vi "LinTabelle zusammenbauen.vi"(8 "error in (no error)":errorcluster caption="Fehler (Eingang, kein Fehler)", 11 "Eingabetabelle":T1) -> (0 "error out":errorcluster caption="Fehler (Ausgang)", 1 "XY-Graph":cluster{dbl[], dbl[]}[](array[cluster]), 2 "Eingabetabelle behandelt":string[][](array[string]), 3 "LIN Ausgabetabelle":string[][](table))   [LabVIEW 2020, in "Linearisierung v2.lvlib"]
uses:
  Linearisierung v2.lvlib
  Eingabetabelle.ctl
panel:
  # "Tabelle:\n0.....Sollwert\n1.....Istwert\n2.....Rohwert\n3.....linearisiert\n4.....abs.Fehler ppm\n5.....Fehler in %\n6.....Deviation\n7.....Temp.Messzelle\n8.....Druck Messzelle\n9.....abs.Fehler ppm linearisiert\n10....Fehler in % linearisiert\n11....abs.Fehler ppm EPA\n12....Fehler in % EPA\n13....abs.Fehler ppm Rohwert\n14....Fehler in % Rohwert"
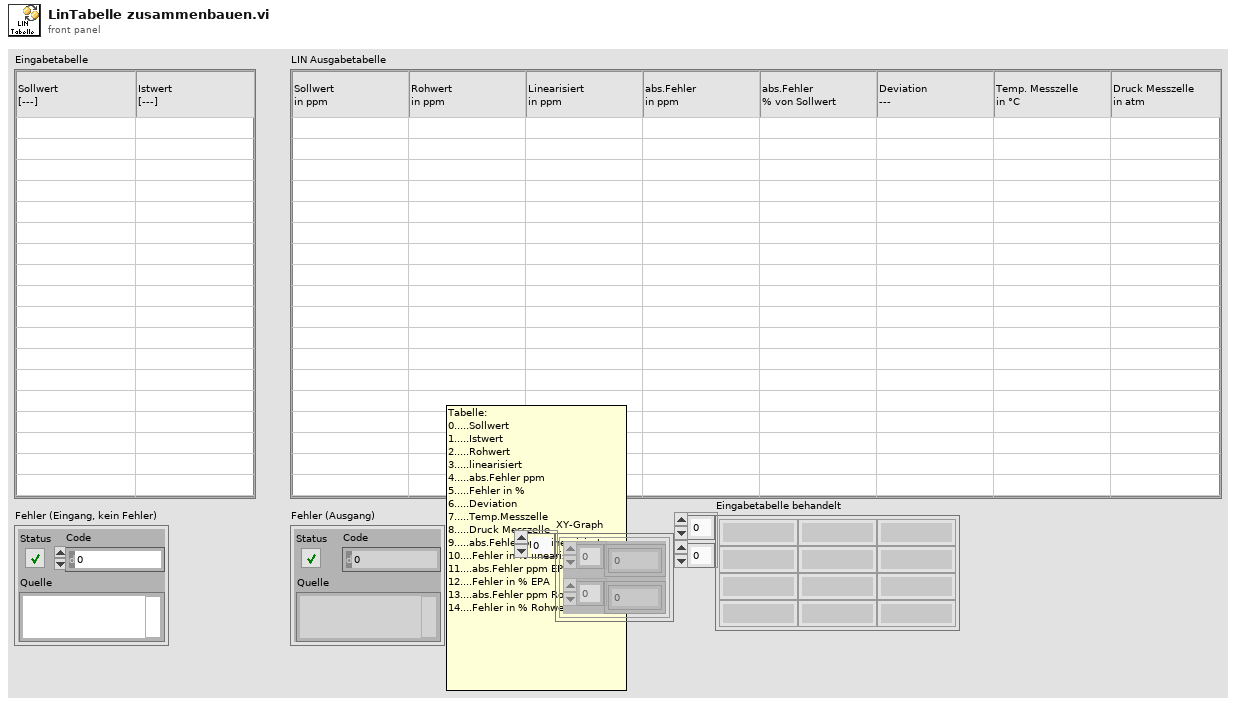
[diagram p1: front panel]
types:
  T1 = typedef "Linearisierung v2.lvlib/Eingabetabelle.ctl" = string[][]
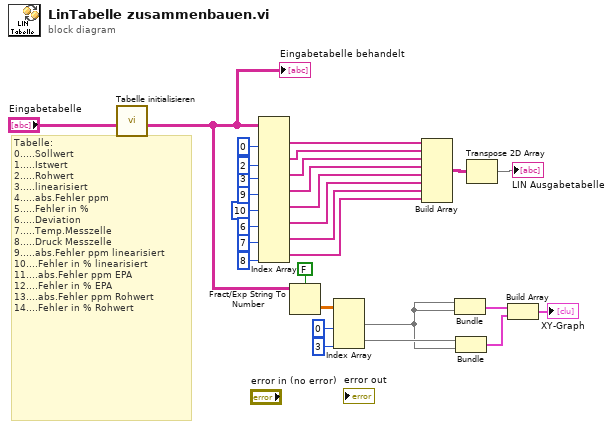
[diagram p0: block diagram]
diagram:
  # "Tabelle:\n0.....Sollwert\n1.....Istwert\n2.....Rohwert\n3.....linearisiert\n4.....abs.Fehler ppm\n5.....Fehler in %\n6.....Deviation\n7.....Temp.Messzelle\n8.....Druck Messzelle\n9.....abs.Fehler ppm linearisiert\n10....Fehler in % linearisiert\n11....abs.Fehler ppm EPA\n12....Fehler in % EPA\n13....abs.Fehler ppm Rohwert\n14....Fehler in % Rohwert"
  n1 = call "Tabelle initialisieren.vi"("Neue Tabelle"="Eingabetabelle") -> ("Tabelle"=w2:string[][])  [unwired: 10 in]
  "Eingabetabelle behandelt" <- w2
  n2 = Index Array(array=w2, index (col) #1=0 ("Deaktivierter Index (Spalte)"), index (col) #2=2 ("Index (Spalte)"), index (col) #3=3 ("Index (Spalte)"), index (col) #4=9 ("Index (Spalte)"), index (col) #5=10 ("Index (Spalte)"), index (col) #6=6 ("Index (Spalte)"), index (col) #7=7 ("Index (Spalte)"), index (col) #8=8 ("Index (Spalte)")) -> (element #1=w29:string[], element #2=w28:string[], element #3=w24:string[], element #4=w21:string[], element #5=w20:string[], element #6=w16:string[], element #7=w15:string[], element #8=w14:string[])  [unwired: 8 in]
  n3 = Fract/Exp String To Number(use system decimal point (T)=FALSE ("Systemdezimalzeichen verwenden (T)"), string=w2) -> (number=w6:dbl[][])  [unwired: 2 in, 1 out]
  n4 = Index Array(array=w6, index (col) #1=0 ("Deaktivierter Index (Spalte)"), index (col) #2=3 ("Index (Spalte)")) -> (element #1=w9:dbl[], element #2=w10:dbl[])  [unwired: 2 in]
  n5 = Build Array(w29, w28, w24, w21, w20, w16, w15, w14) -> (w13:string[][])
  n6 = Bundle(w9, w9) -> (w4:cluster{dbl[], dbl[]})  [unwired: 1 in]
  n7 = Bundle(w10, w9) -> (w5:cluster{dbl[], dbl[]})  [unwired: 1 in]
  n8 = Transpose 2D Array(2D array=w13) -> (transposed array=→"LIN Ausgabetabelle":string[][])
  n9 = Build Array(w4, w5) -> (→"XY-Graph":cluster{dbl[], dbl[]}[])
